vi "ADCP_Get_Error_And_Status.vi"(8 "error in (no error)":errorcluster, 10 "Node ID":i32=-1, 11 "ADCP In":refnum<class "ADCP.lvclass">) -> (0 "error out":errorcluster, 2 "Error and Status":T1, 3 "ADCP Out":refnum<class "ADCP.lvclass">)   [LabVIEW 2017, in "ADCP.lvclass"]
uses:
  ADCP.lvclass
  ADCP.lvclass/ADCP.ctl
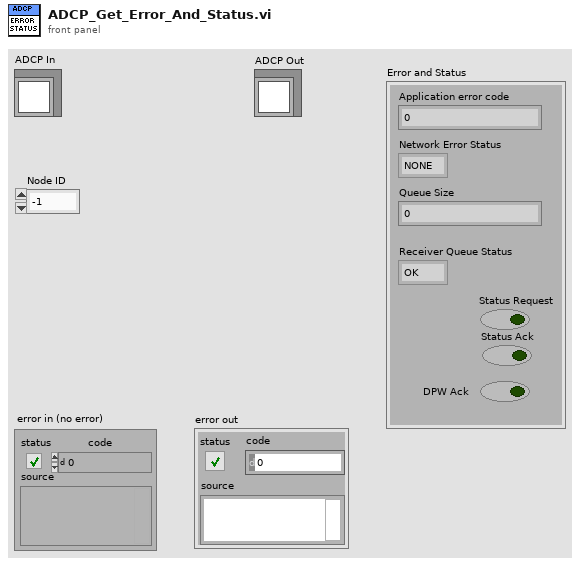
[diagram p1: front panel]
types:
  T1 = cluster{"Application error code":u16, "Network Error Status":enum16{"NONE", "CONNECTION_ALREADY_OPEN", "CONNECTION_ALREADY_CLOSED", "INVALID_FRAME_REQUEST"}, "Queue Size":u16, "Receiver Queue Status":enum16{"OK", "EMPTY", "FULL"}, "Status Request":bool, "Status Ack":bool, "DPW Ack":bool}
  T2 = cluster{"Application error code":u16, "Network Error Status":enum16{"NONE", "CONNECTION_ALREADY_OPEN", "CONNECTION_ALREADY_CLOSED", "INVALID_FRAME_REQUEST"}, "Queue Size":u16, "Receiver Queue Status":enum16{"OK", "EMPTY", "FULL"}, "Status Request":bool, "Status Ack":bool, "WDP Ack":bool}
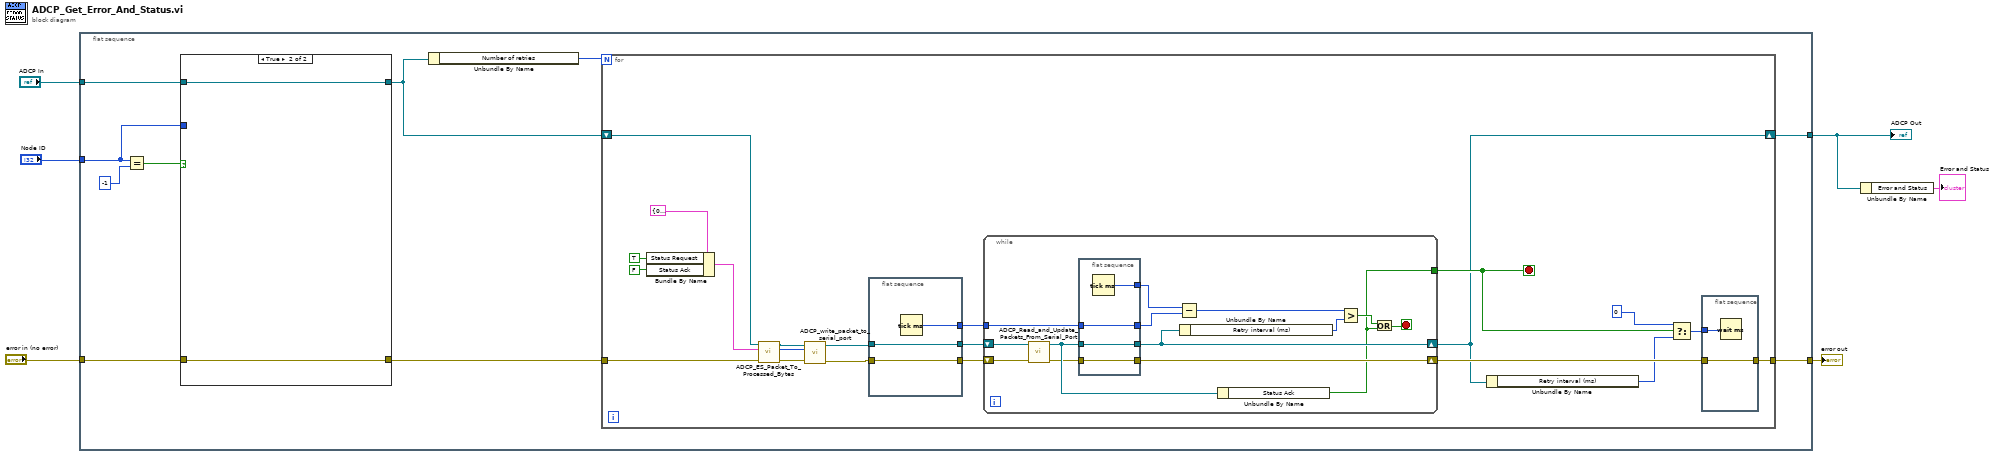
[diagram p0: block diagram]
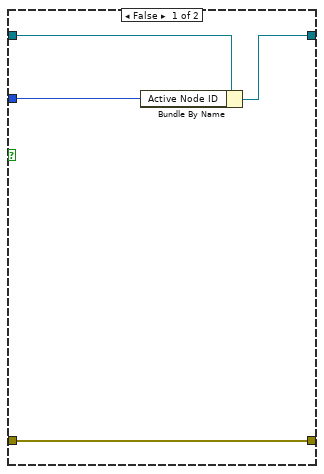
[diagram p2: hidden frame]
diagram:
  n1 = flat-sequence {
    tunnel: "ADCP In" -> [w13]
    tunnel: "error in (no error)" -> [w15]
    tunnel: "Node ID" -> [w12]
    tunnel: [w8] -> w2
    tunnel: [w7] -> w3
    frame #0 {
      n2 = Equal?(x=w12, y=-1) -> (x = y?=w14:bool)
      n3 = case shown="True" w14 {
        tunnel: w15 -> [w61 w65]
        tunnel: w13 -> [w64 w66]
        tunnel: [w62 w66] -> w9
        tunnel: w12 -> [w63 _]
        tunnel: [w61 w65] -> w11
        frame False {
          n4 = Bundle By Name(cluster=w64, "Active Node ID"=w63) -> (w62:refnum<class "ADCP.lvclass">)
        }
        frame True {
        }
      }
      n5 = Unbundle By Name(w9) -> ("Number of retries"=w10:u16)
      n6 = for {
        N: w10 -> [_]
        tunnel: w11 -> [w37]
        shift-right: [w28] -> w8
        shift-left: w9 -> [w36]
        tunnel: [w26] -> w7
        stop <- w31 stop-if-true
        n7 = Bundle By Name(cluster=T1 {"Application error code"=0, "Network Error Status"=enum."NONE", "Queue Size"=0, "Receiver Queue Status"=enum."OK", "Status Request"=FALSE, "Status Ack"=FALSE, "DPW Ack"=FALSE} ("ADCP Error and Status Packet"), "Status Request"=TRUE, "Status Ack"=FALSE) -> (w20:T1)
        n8 = call "ADCP_ES_Packet_To_Processed_Bytes.vi"("error in (no error)"=w37, "ES Packet In"=w20, "ADCP In"=w36) -> ("error out"=w23:errorcluster, "Processed Packet Bytes"=w25:u8[], "ADCP Out"=w24:refnum<class "ADCP.lvclass">)  [unwired: 6 in]
        n9 = call "ADCP_write_packet_to_serial_port.vi"("error in (no error)"=w23, "Packet Bytes"=w25, "ADCP In"=w24) -> ("error out"=w22:errorcluster, "ADCP Out"=w21:refnum<class "ADCP.lvclass">)  [unwired: 7 in]
        n10 = flat-sequence {
          tunnel: w21 -> [w42]
          tunnel: [w42] -> w35
          tunnel: w22 -> [w41]
          tunnel: [w41] -> w34
          tunnel: [w40] -> w33
          frame #0 {
            n11 = Tick Count (ms)() -> (millisecond timer value=w40:u32)
          }
        }
        n12 = while {
          shift-right: [w47] -> w28
          shift-left: w35 -> [w55]
          shift-right: [w52] -> w32
          shift-left: w34 -> [w56]
          tunnel: w33 -> [w50]
          tunnel: [w43] -> w31
          stop <- w44 stop-if-true
          n13 = call "ADCP_Read_and_Update_Packets_From_Serial_Port.vi"("error in (no error)"=w56, "ADCP In"=w55) -> ("error out"=w53:errorcluster, "ADCP out"=w54:refnum<class "ADCP.lvclass">)  [unwired: 6 in, 2 out]
          n14 = flat-sequence {
            tunnel: w54 -> [w60]
            tunnel: [w60] -> w47
            tunnel: w53 -> [w59]
            tunnel: [w59] -> w52
            tunnel: [w58] -> w51
            tunnel: w50 -> [w57]
            tunnel: [w57] -> w49
            frame #0 {
              n15 = Tick Count (ms)() -> (millisecond timer value=w58:u32)
            }
          }
          n16 = Subtract(x=w51, y=w49) -> (x-y=w48:u32)
          n17 = Unbundle By Name(w47) -> ("Retry interval (ms)"=w46:u16)
          n18 = Unbundle By Name(w54) -> ("Status Ack"=w43:bool)
          n19 = Greater?(x=w48, y=w46) -> (0:w45:bool)
          n20 = Or(x=w45, y=w43) -> (x .or. y?=w44:bool)
        }
        n21 = Unbundle By Name(w28) -> ("Retry interval (ms)"=w27:u16)
        n22 = Select(t=0, s=w31, f=w27) -> (s? t:f=w29:i32)
        n23 = flat-sequence {
          tunnel: w32 -> [w39]
          tunnel: [w39] -> w26
          tunnel: w29 -> [w38]
          frame #0 {
            n24 = Wait (ms)(milliseconds to wait=w38) -> ()  [unwired: 1 out]
          }
        }
      }
    }
  }
  n25 = Unbundle By Name(w2) -> ("Error and Status"=→"Error and Status":T2)
  "ADCP Out" <- w2
  "error out" <- w3
